vi "Get Temperature.vi"(8 "Error In":errorcluster, 11 "ECU COM Port":refnum<visa-resource-name>) -> (0 "Error Out":errorcluster, 1 "Temp (string)":string, 2 "Temp (double)":dbl, 3 "ECU COM Port Out":refnum<visa-resource-name>)   [LabVIEW 2017]
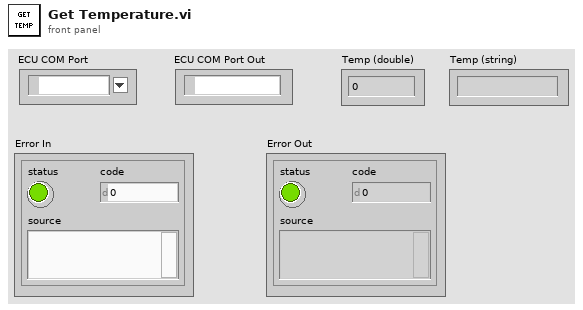
[diagram p1: front panel]
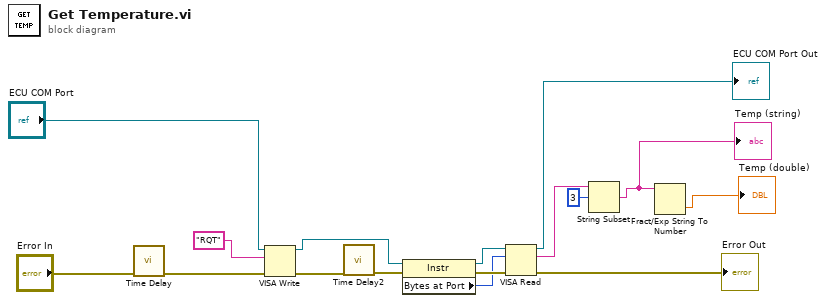
[diagram p0: block diagram]
diagram:
  n1 = call "Time Delay"("error in (no error)"="Error In") -> ("error out"=w13:errorcluster)  [unwired: 10 in]
  n2 = VISA Write(VISA resource name="ECU COM Port", write buffer="RQT", error in (no error)=w13) -> (VISA resource name out=w6:refnum<visa-resource-name>, error out=w12:errorcluster)  [unwired: 1 out]
  n3 = call "Time Delay2"("error in (no error)"=w12) -> ("error out"=w8:errorcluster)  [unwired: 10 in]
  n4 = property class="Instr"(reference=w6, error in=w8) -> (reference out=w11:refnum<visa-resource-name>, error out=w10:errorcluster, "Bytes at Port"=w9:u32)
  n5 = VISA Read(VISA resource name=w11, byte count=w9, error in (no error)=w10) -> (VISA resource name out=→"ECU COM Port Out":refnum<visa-resource-name>, read buffer=w4:string, error out=→"Error Out":errorcluster)  [unwired: 1 out]
  n6 = String Subset(string=w4, offset (0)=3) -> (substring=w1:string)  [unwired: 1 in]
  "Temp (string)" <- w1
  n7 = Fract/Exp String To Number(string=w1) -> (number=→"Temp (double)":dbl)  [unwired: 3 in, 1 out]
